vi "扫码触发.vi"(8 "error in (no error)":errorcluster caption="错误输入（无错误）", 9 "超时秒数":dbl, 10 "远程端口或服务名称":u16=51236, 11 "地址":string="192.168.3.100") -> (0 "error out 2":errorcluster caption="错误输出", 2 "结果":bool, 3 "数据输出":string)   [LabVIEW 2017]
uses:
  <vilib>/Instr/_visa.llb/VISA Configure Serial Port (Instr).vi
panel:
  in  "时间":dbl
  out "BOXID":string
  out "result":bool
  out "error out":errorcluster caption="错误输出"
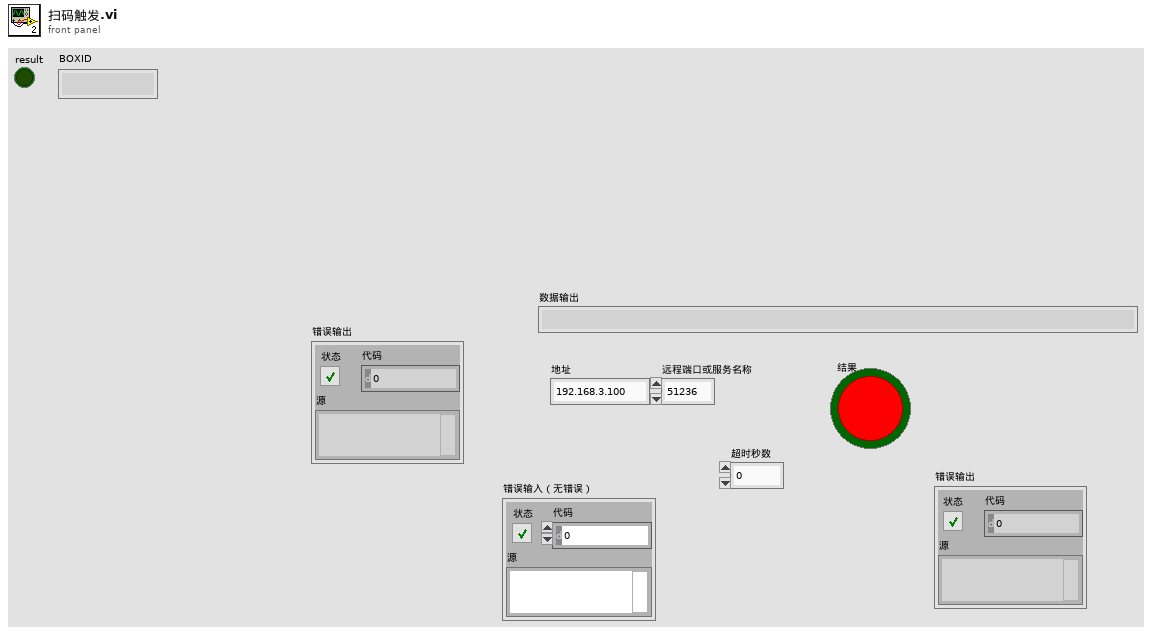
[diagram p1: front panel]
types:
  T1 = enum16{"Standard", "Buffered", "CRLF", "Immediate"}
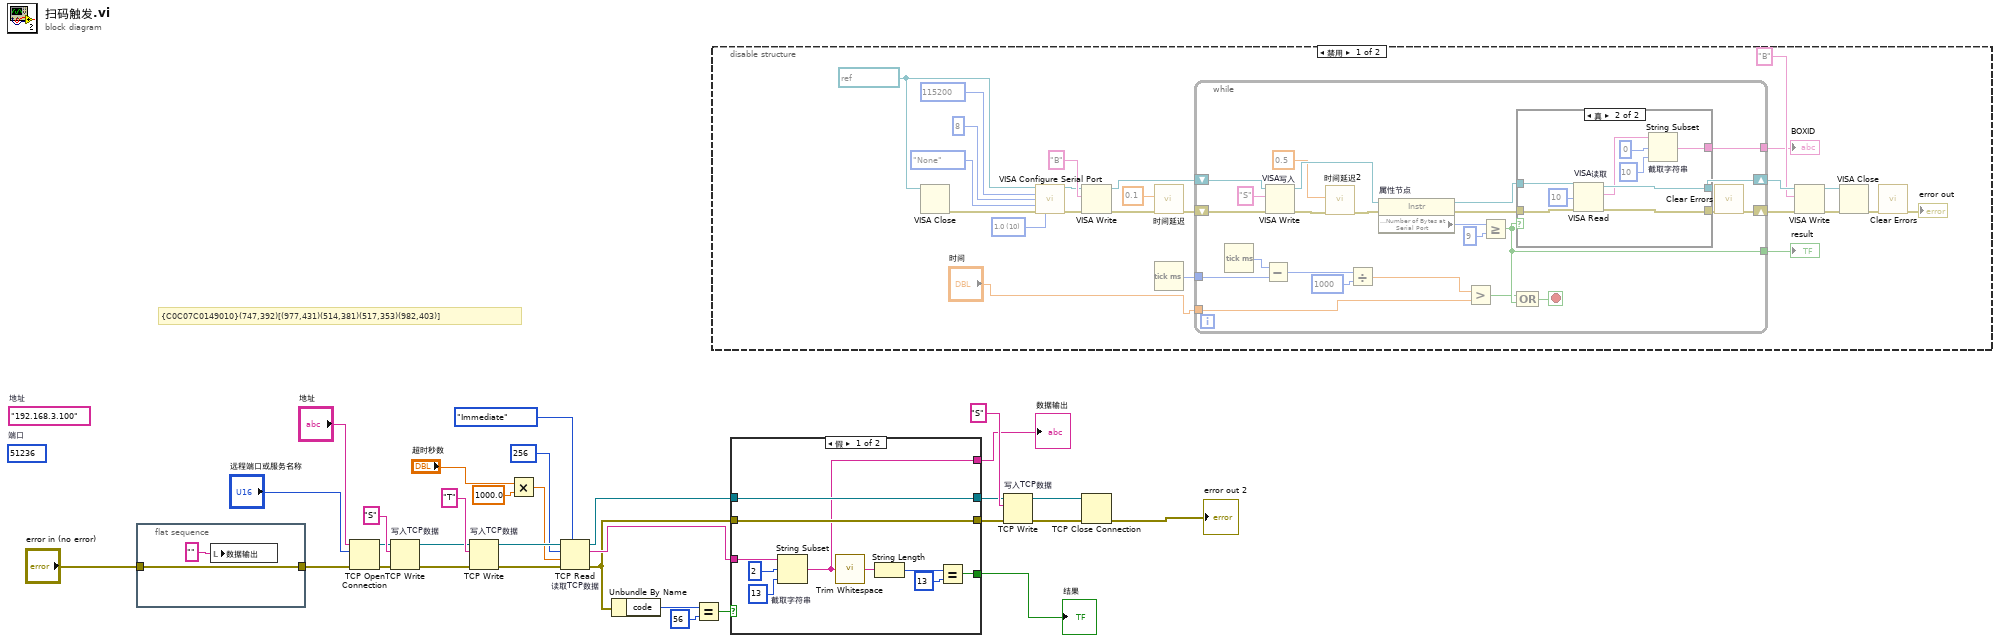
[diagram p0: block diagram]
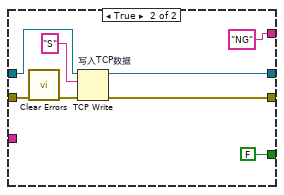
[diagram p2: hidden frame]
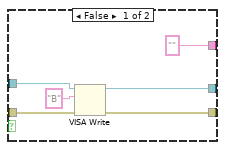
[diagram p3: hidden frame]
diagram:
  (unwired) u16 51236  # 端口
  (unwired) "192.168.3.100"  # 地址
  # "{C0C07C0149010}(747,392)[(977,431)(514,381)(517,353)(982,403)]"
  n1 = flat-sequence {
    tunnel: "error in (no error)" -> [w33]
    tunnel: [w33] -> w1
    frame #0 {
      n2 = local write "数据输出"("" ("数据输出")) -> ()
    }
  }
  n3 = TCP Open Connection(address="地址", remote port or service name="远程端口或服务名称", error in (no error)=w1) -> (connection ID=w6:refnum<k5>, error out=w7:errorcluster)  [unwired: 2 in]
  n4 = TCP Write "写入TCP数据"(connection ID=w6, data in="S" ("数据输入"), error in (no error)=w7) -> (connection ID out=w5:refnum<k5>, error out=w4:errorcluster)  [unwired: 2 out]
  n5 = TCP Write "写入TCP数据"(connection ID=w5, data in="T" ("数据输入"), error in (no error)=w4) -> (connection ID out=w30:refnum<k5>, error out=w29:errorcluster)  [unwired: 2 out]
  n6 = Multiply(x="超时秒数", y=1000.0) -> (x*y=w13:dbl)
  n7 = TCP Read "读取TCP数据"(connection ID=w30, bytes to read=256 ("读取的字节"), error in (no error)=w29, 7:T1."Immediate" ("模式（标准）"), 9:w13) -> (connection ID out=w17:refnum<k5>, data out=w16:string, error out=w12:errorcluster)
  n8 = Unbundle By Name(w12) -> ("code"=w11:i32)
  n9 = Equal?(x=w11, y=56) -> (x = y?=w9:bool)
  n10 = disable-structure shown="禁用" {
    frame Disabled {
      w52 = u16 10 items=["1.0"=10, "1.5"=15, "2.0"=20] ("stop bits (10: 1 bit)")
      w51 = refnum<visa-resource-name> "COM1" ("VISA resource name")
      n11 = VISA Close(VISA resource name=w51) -> (error out=w50:errorcluster)  [unwired: 1 in]
      n12 = call-poly "VISA Configure Serial Port"("VISA resource name"=w51, "baud rate (9600)"=u32 115200, "data bits (8)"=u16 8, "parity (0:none)"=enum16{"None", "Odd", "Even", "Mark", "Space"}."None", "error in (no error)"=w50, "stop bits (10: 1 bit)"=w52) -> ("VISA resource name out"=w47:refnum<visa-resource-name>, "error out"=w48:errorcluster)  [unwired: 8 in]
      n13 = VISA Write(VISA resource name=w47, write buffer="B" ("写入缓冲区"), error in (no error)=w48) -> (VISA resource name out=w46:refnum<visa-resource-name>, error out=w45:errorcluster)  [unwired: 1 out]
      n14 = call "时间延迟"("error in (no error)"=w45, "Delay Time (s)"=0.1) -> ("error out"=w44:errorcluster)  [unwired: 9 in]
      n15 = Tick Count (ms)() -> (millisecond timer value=w35:u32)
      n16 = while {
        tunnel: [w77] -> w39
        tunnel: [w76] -> w36
        shift-right: [w81] -> w57
        shift-left: w46 -> [w79]
        shift-right: [w80] -> w56
        shift-left: w44 -> [w78]
        tunnel: w35 -> [w62]
        tunnel: "时间" -> [w58]
        stop <- w75 stop-if-true
        n17 = Tick Count (ms)() -> (millisecond timer value=w63:u32)
        n18 = Subtract(x=w63, y=w62) -> (x-y=w61:u32)
        n19 = VISA Write "VISA写入"(VISA resource name=w79, write buffer="S" ("写入缓冲区"), error in (no error)=w78) -> (VISA resource name out=w72:refnum<visa-resource-name>, error out=w67:errorcluster)  [unwired: 1 out]
        n20 = call "时间延迟2"("error in (no error)"=w67, "Delay Time (s)"=0.5) -> ("error out"=w66:errorcluster)  [unwired: 9 in]
        n21 = Divide(x=w61, y=u32 1000) -> (x/y=w59:dbl)
        n22 = property on="属性节点" class="Instr"(reference=w72, error in=w66) -> (reference out=w71:refnum<visa-resource-name>, error out=w65:errorcluster, "Serial Settings:Number of Bytes at Serial Port"=w70:u32)
        n23 = Greater?(x=w59, y=w58) -> (0:w74:bool)
        n24 = Greater Or Equal?(x=w70, y=u32 9) -> (x >= y?=w76:bool)
        n25 = case shown="真" w76 {
          tunnel: [w84 w96] -> w81
          tunnel: w71 -> [w86 w95]
          tunnel: w65 -> [w85 w94]
          tunnel: ["" ("read buffer") w93] -> w77
          tunnel: [w83 w88] -> w68
          frame False {
            n26 = VISA Write(VISA resource name=w86, write buffer="B" ("写入缓冲区"), error in (no error)=w85) -> (VISA resource name out=w84:refnum<visa-resource-name>, error out=w83:errorcluster)  [unwired: 1 out]
          }
          frame True {
            n27 = VISA Read "VISA读取"(VISA resource name=w95, byte count=u32 10 ("字节总数"), error in (no error)=w94) -> (VISA resource name out=w96:refnum<visa-resource-name>, read buffer=w92:string, error out=w88:errorcluster)  [unwired: 1 out]
            n28 = String Subset "截取字符串"(string=w92, offset (0)=0, length (rest)=10 ("length (rest)")) -> (substring=w93:string)
          }
        }
        n29 = Compound Arithmetic op=OR(w74, w76) -> (w75:bool)
        n30 = call <vilib>:"Clear Errors.vi"("error in (no error)"=w68) -> ("error out"=w80:errorcluster)  [unwired: 5 in, 1 out]
      }
      "result" <- w36
      "BOXID" <- w39
      n31 = VISA Write(VISA resource name=w57, write buffer="B" ("写入缓冲区"), error in (no error)=w56) -> (VISA resource name out=w41:refnum<visa-resource-name>, error out=w42:errorcluster)  [unwired: 1 out]
      n32 = VISA Close(VISA resource name=w41, error in (no error)=w42) -> (error out=w38:errorcluster)
      n33 = call <vilib>:"Clear Errors.vi"("error in (no error)"=w38) -> ("error out"=→"error out":errorcluster)  [unwired: 5 in, 1 out]
    }
    frame Enabled {
    }
  }
  n34 = case shown="假" w9 {
    tunnel: [w101 "NG" ("data out")] -> w20
    tunnel: w16 -> [w104 _]
    tunnel: w17 -> [w103 w113]
    tunnel: [w103 w112] -> w24
    tunnel: w12 -> [w102 w111]
    tunnel: [w102 w110] -> w25
    tunnel: [w97 FALSE] -> w3
    frame False {
      n35 = String Subset "截取字符串"(string=w104, offset (0)=2, length (rest)=13 ("length (rest)")) -> (substring=w101:string)
      n36 = call <vilib>:"Trim Whitespace.vi"("string"=w101) -> ("trimmed string"=w98:string)  [unwired: 1 in]
      n37 = String Length(string=w98) -> (length=w100:i32)
      n38 = Equal?(x=w100, y=13) -> (x = y?=w97:bool)
    }
    frame True {
      n39 = call <vilib>:"Clear Errors.vi"("error in (no error)"=w111) -> ("error out"=w107:errorcluster)  [unwired: 5 in, 1 out]
      n40 = TCP Write "写入TCP数据"(connection ID=w113, data in="S", error in (no error)=w107) -> (connection ID out=w112:refnum<k5>, error out=w110:errorcluster)  [unwired: 2 out]
    }
  }
  "数据输出" <- w20
  "结果" <- w3
  n41 = TCP Write "写入TCP数据"(connection ID=w24, data in="S", error in (no error)=w25) -> (connection ID out=w28:refnum<k5>, error out=w27:errorcluster)  [unwired: 2 out]
  n42 = TCP Close Connection(connection ID=w28, error in (no error)=w27) -> (error out=→"error out 2":errorcluster)  [unwired: 1 in, 1 out]
